vi "Decode.vi"(10 "Wire Type":T2, 11 "Buffer":u8[](array[numeric]) format="%.0x") -> (2 "error out":errorcluster, 3 "Data":T1)   [LabVIEW 2020, in "StartSeq.lvlib"]
uses:
  StartSeq.lvlib
  lv-protoc/LV-Proto/Wire Type.ctl
  Data.ctl
  lv-protoc/LV-Proto/LV-Proto.lvlib
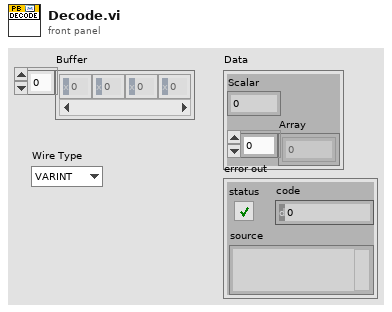
[diagram p1: front panel]
types:
  T1 = typedef "StartSeq.lvlib/Data.ctl" = cluster{"Scalar":dbl, "Array":dbl[]}
  T2 = typedef "LV-Proto.lvlib/Wire Type.ctl" = enum8{"VARINT", "I64", "LEN", "SGROUP (Deprecated)", "EGROUP (Deprecated)", "I32"}
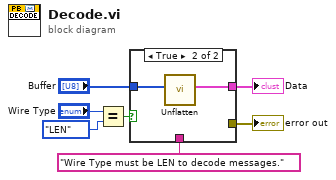
[diagram p0: block diagram]
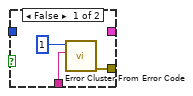
[diagram p2: hidden frame]
diagram:
  n1 = Equal?(x="Wire Type", y=Wire_Type."LEN") -> (x = y?=w6:bool)
  n2 = case shown="True" w6 {
    tunnel: "Buffer" -> [_ w12]
    tunnel: [w9 _] -> w4
    tunnel: "Wire Type must be LEN to decode messages." -> [w8 _]
    tunnel: [_ w11] -> w3
    frame False {
      n3 = call <vilib>:"Error Cluster From Error Code.vi"("error message (\"\")"=w8, "error code (0)"=1) -> ("error out"=w9:errorcluster)  [unwired: 7 in]
    }
    frame True {
      n4 = call "Unflatten.vi"("Buffer"=w12) -> ("Data"=w11:T1)  [unwired: 9 in, 1 out]
    }
  }
  "Data" <- w3
  "error out" <- w4
